vi "Create.vi"(0 "rx output divider":T1, 5 "horizontal step size":i16=2, 7 "vertical step size":i16=2, 11 "error in":errorcluster) -> (4 "eye scan point iterator out":refnum<class "niHighSpeedSerial Rectangular Eye Scan Point Iterator v1 Host.lvclass">, 15 "error out":errorcluster)   [LabVIEW 2014, in "niHighSpeedSerial Rectangular Eye Scan Point Iterator v1 Host.lvclass"]
doc: "Creates a Point Iterator object.\n\n<B>Input Parameters</B>\n\n<B>rx output divider</B> represents the configuration of the receiver output divider. This should match the values configured with RXRATE and RXOUT_DIV.\nenum values: 1,2,4,8,16\n\n<B>horizontal step size</B> is the number of offsets to skip between each point on the horizontal axis.\n\n<B>vertical step size</B> is the number of offsets to skip between each point on the vertical axis.\n\n<B>error in</B> describes error conditions that occur before this node runs. This input provides standard 'error in' functionality.\n\n<B>Output Parameters</B>\n\n<B>eye scan point iterator out</B> is the outgoing wire for the Eye Scan Point Iterator class object\n\n<B>error out</B> contains error information. This output provides standard 'error out' functionality."
uses:
  <instrlib>/niHighSpeedSerial/Eye Scan/v1/Host/Impl/Rect Iter/niHighSpeedSerial Rectangular Eye Scan Point Iterator v1 Host.lvclass
  <instrlib>/niHighSpeedSerial/Eye Scan/v1/Host/Common/Public/RX Output Divider.ctl
  <instrlib>/niHighSpeedSerial/Eye Scan/v1/Host/Impl/Rect Iter/niHighSpeedSerial Rectangular Eye Scan Point Iterator v1 Host.lvclass/niHighSpeedSerial Rectangular Eye Scan Point Iterator v1 Host.ctl
  <instrlib>/niHighSpeedSerial/Eye Scan/v1/Host/Impl/Eye Scan Point Iterator/niHighSpeedSerial Eye Scan Point Iterator v1 Host.lvclass
  <instrlib>/niHighSpeedSerial/Eye Scan/v1/Host/Common/niHighSpeedSerial Eye Scan Common v1 Host.lvlib
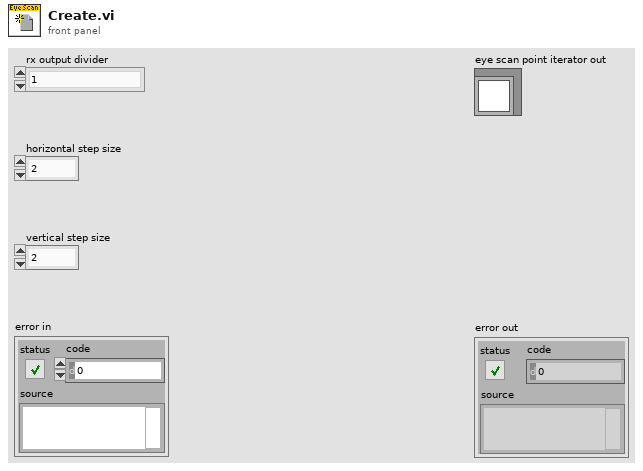
[diagram p1: front panel]
types:
  T1 = typedef "niHighSpeedSerial Eye Scan Common v1 Host.lvlib/RX Output Divider.ctl" = enum16{"1", "2", "4", "8", "16"}
  T2 = typedef "niHighSpeedSerial Eye Scan Common v1 Host.lvlib/Point.ctl" = cluster{"point offsets":T3, "sample count":u64, "error count":u64, "bit error rate":dbl}
  T3 = typedef "niHighSpeedSerial Eye Scan Common v1 Host.lvlib/Point Offsets.ctl" = cluster{"horizontal offset":i16, "vertical offset":i8}
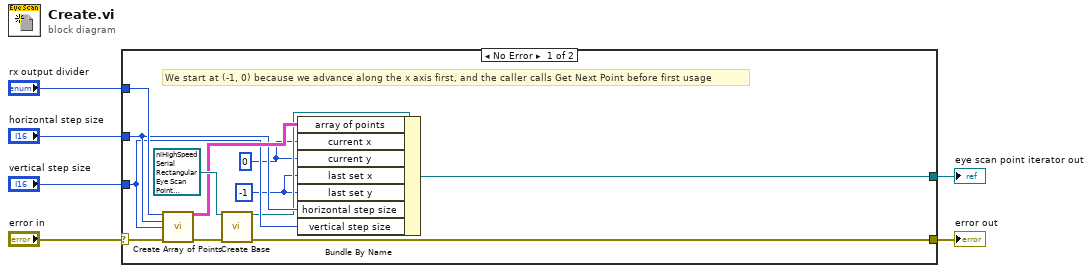
[diagram p0: block diagram]
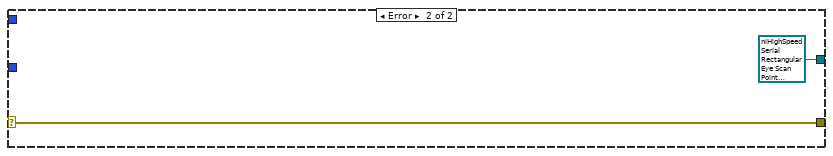
[diagram p2: hidden frame]
diagram:
  n1 = case shown="No Error" "error in" {
    selector: "error in" -> [w15 w20]
    tunnel: [w17 w20] -> w5
    tunnel: [w9 refnum<class "niHighSpeedSerial Rectangular Eye Scan Point Iterator v1 Host.lvclass"> refnum ("Rectangular Eye Scan Point Iterator.lvclass 2")] -> w4
    tunnel: "horizontal step size" -> [w12 _]
    tunnel: "vertical step size" -> [w11 _]
    tunnel: "rx output divider" -> [w16 _]
    frame No Error {
      w7 = -1 ("y")
      w8 = 0 ("x")
      # "We start at (-1, 0) because we advance along the x axis first, and the caller calls Get Next Point before first usage"
      n2 = call <instrlib>:"Create Array of Points.vi"("rx output divider"=w16, "horizontal step size"=w12, "vertical step size"=w11, "error in"=w15) -> ("array of points"=w13:T2[][], "error out"=w14:errorcluster)  [unwired: 10 in]
      n3 = call <instrlib>:"Create Base.vi"("eye scan point iterator"=refnum<class "niHighSpeedSerial Rectangular Eye Scan Point Iterator v1 Host.lvclass"> refnum ("Rectangular Eye Scan Point Iterator.lvclass 2"), "error in"=w14) -> ("eye scan point iterator out"=w10:refnum<class "niHighSpeedSerial Rectangular Eye Scan Point Iterator v1 Host.lvclass">, "error out"=w17:errorcluster)  [unwired: 12 in]
      n4 = Bundle By Name(cluster=w10, "array of points"=w13, "current x"=w8, "current y"=w8, "last set x"=w7, "last set y"=w7, "horizontal step size"=w12, "vertical step size"=w11) -> (w9:refnum<class "niHighSpeedSerial Rectangular Eye Scan Point Iterator v1 Host.lvclass">)
    }
    frame Error {
    }
  }
  "eye scan point iterator out" <- w4
  "error out" <- w5
